vi "datasetName.get.vi"(8 "error in (no error)":errorcluster, 11 "dataset in":refnum<class "dataset.lvclass">) -> (0 "error out":errorcluster, 2 "datasetName":string, 3 "dataset out":refnum<class "dataset.lvclass">)   [LabVIEW 2020, in "datasources.lvlib" / "dataset.lvclass"]
uses:
  dataset.lvclass
  dataset.lvclass/dataset.ctl
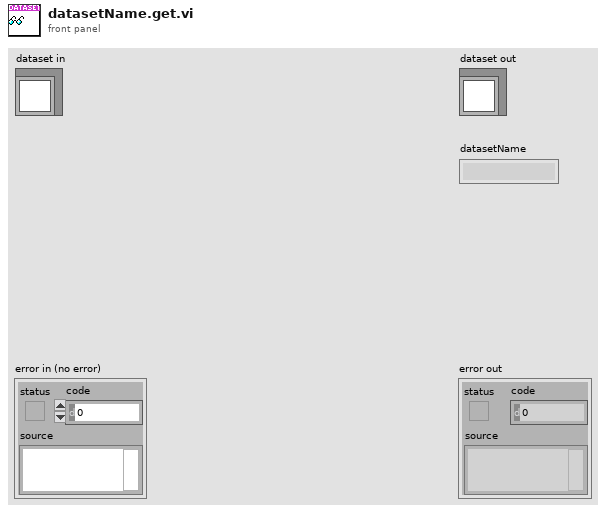
[diagram p1: front panel]
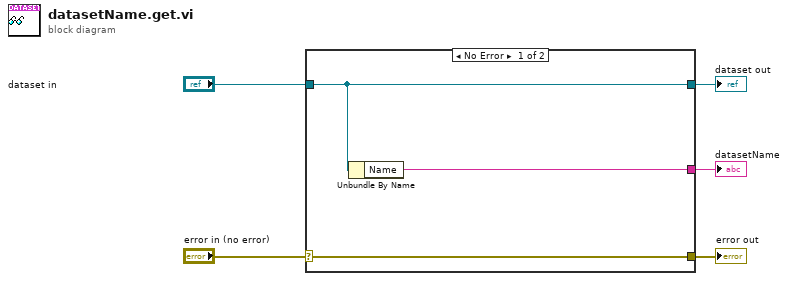
[diagram p0: block diagram]
diagram:
  n1 = case shown="No Error" "error in (no error)" {
    selector: "error in (no error)" -> [w8 w9]
    tunnel: [w8 w9] -> w4
    tunnel: [w7 w10] -> w2
    tunnel: "dataset in" -> [w7 w10]
    tunnel: [w6 _] -> w1
    frame No Error {
      n2 = Unbundle By Name(w7) -> ("Name"=w6:string)
    }
    frame Error {
    }
  }
  "error out" <- w4
  "dataset out" <- w2
  "datasetName" <- w1
